vi "WeatherReportTestsForEXE.vi"(8 "error in (no error)":errorcluster, 10 "Drona Tests PPL":path, 11 "EXE Path":path) -> (0 "error out":errorcluster)   [LabVIEW 2016]
uses:
  Drona.lvlib
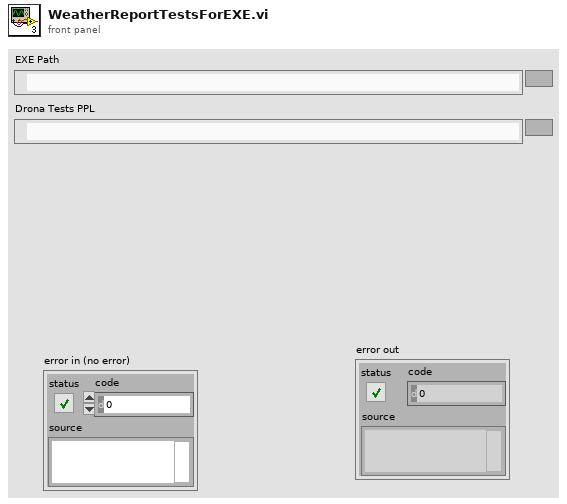
[diagram p1: front panel]
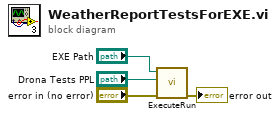
[diagram p0: block diagram]
diagram:
  n1 = call "ExecuteRun.vi"("error in (no error)"="error in (no error)", "Drona Tests PPL"="Drona Tests PPL", "EXE Path"="EXE Path") -> ("error out"=→"error out":errorcluster)  [unwired: 8 in]
